vi "getChipSize.vi"(6 "Delay between send and receive [ms]":i32=100, 8 "error in (no error)":errorcluster, 11 "CCD in":refnum<class "CCD.lvclass">) -> (0 "error out":errorcluster, 1 "chip size, y":i32, 2 "chip size, x":i32, 3 "CCD out":refnum<class "CCD.lvclass">)   [LabVIEW 2023, in "CCD.lvclass"]
uses:
  CCD.lvclass
  Chipsize.ctl
  acd18d44-655d-42a0-b073-c3a6adbe6448.vi
  91ff1499-e288-40ed-a9bd-2102f7a68490.vi
  <vilib>/JDP Science/JSONtext/Variant to JSON Text.vi
  <vilib>/JDP Science/JSONtext/Set Item.vi
  <vilib>/JDP Science/JSONtext/JSON text to Variant.vi
  <vilib>/JDP Science/JSONtext/LVClass Serializer/JSONtext LVClass Serializer.lvclass
  CCD.lvclass/CCD.ctl
  GenericDevice/GenericDevice.lvclass
  <vilib>/IlluminatedG/lv-web-crypto/lv-json/JSON/JSON.lvlib
panel:
  # "Connector Pane"
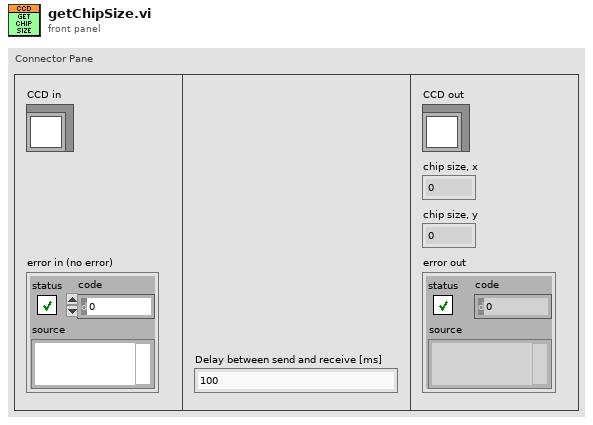
[diagram p1: front panel]
types:
  T1 = typedef "CCD.lvclass/Chipsize.ctl" = cluster{"x":i32, "y":i32}
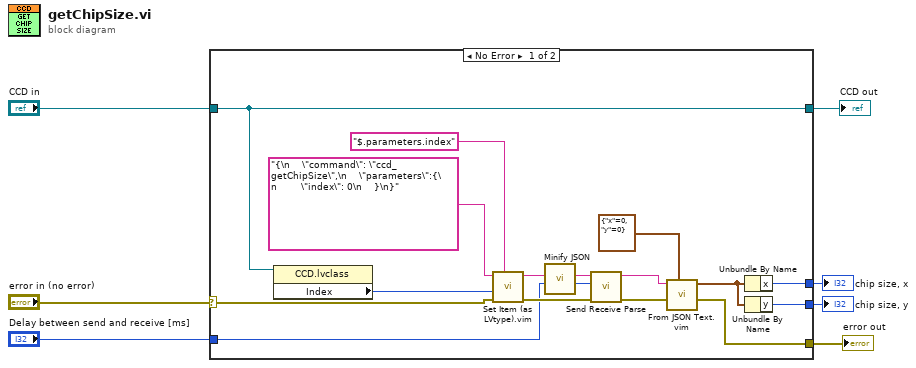
[diagram p0: block diagram]
diagram:
  n1 = case shown="No Error" "error in (no error)" {
    selector: "error in (no error)" -> [w19 w25]
    tunnel: [w18 w25] -> w6
    tunnel: [w21 w24] -> w4
    tunnel: "CCD in" -> [w21 w24]
    tunnel: [w12 _] -> w3
    tunnel: [w11 _] -> w2
    tunnel: "Delay between send and receive [ms]" -> [w8 _]
    frame No Error {
      n2 = property class="CCD.lvclass"(reference=w21) -> ("Index"=w20:i32)  [unwired: 1 in, 2 out]
      n3 = call "Set Item (as LVtype).vim"("$Path or Item Name"="$.parameters.index", "error in (no error)"=w19, "Anything"=w20, "JSON"="{\n    \"command\": \"ccd_getChipSize\",\n    \"parameters\":{\n        \"index\": 0\n    }\n}") -> ("error out"=w15:errorcluster, "<JSON>"=w10:string)  [unwired: 4 in, 1 out]
      n4 = call <vilib>:"Minify JSON.vi"("JSON String"=w10) -> ("Minified JSON"=w9:string)  [unwired: 10 in]
      n5 = call "Send Receive Parse.vi"("error in"=w15, "Delay between send and receive [ms]"=w8, "<JSON>"=w9) -> ("error out"=w14:errorcluster, "results-JSON string"=w16:string)  [unwired: 6 in, 1 out]
      n6 = call "From JSON Text.vim"("Data Type and Default Value"=T1 {"x"=0, "y"=0} ("Chipsize"), "error in (no error)"=w14, "JSON"=w16) -> ("error out"=w18:errorcluster, "Data out"=w13:T1)  [unwired: 7 in]
      n7 = Unbundle By Name(w13) -> ("x"=w12:i32)
      n8 = Unbundle By Name(w13) -> ("y"=w11:i32)
    }
    frame Error {
    }
  }
  "error out" <- w6
  "CCD out" <- w4
  "chip size, x" <- w3
  "chip size, y" <- w2
